vi "TCP Send Synchronous Request.vi"(8 "error in (no error)":errorcluster, 10 "Request String in":string) -> (0 "error out":errorcluster, 2 "Response":string)   [LabVIEW 2015]
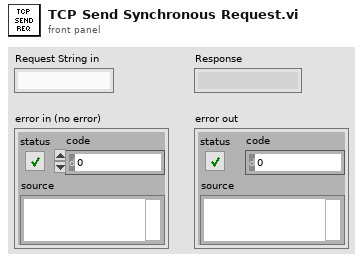
[diagram p1: front panel]
types:
  T1 = enum16{"Standard", "Buffered", "CRLF", "Immediate"}
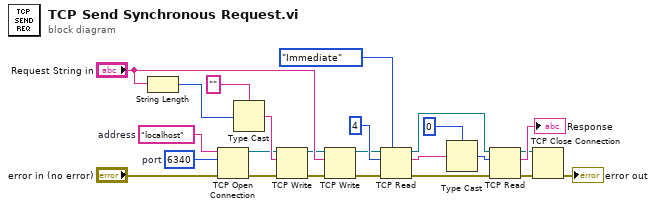
[diagram p0: block diagram]
diagram:
  w3 = u16 6340  # port
  w2 = "localhost"  # address
  n1 = String Length(string="Request String in") -> (length=w12:i32)
  n2 = TCP Open Connection(address=w2, remote port or service name=w3, error in (no error)="error in (no error)") -> (connection ID=w7:refnum<k5>, error out=w9:errorcluster)  [unwired: 2 in]
  n3 = Type Cast(type="" ("format string"), x=w12) -> (*(type *) &x=w11:string)
  n4 = TCP Write(connection ID=w7, data in=w11, error in (no error)=w9) -> (connection ID out=w8:refnum<k5>, error out=w10:errorcluster)  [unwired: 1 in, 1 out]
  n5 = TCP Write(connection ID=w8, data in="Request String in", error in (no error)=w10) -> (connection ID out=w4:refnum<k5>, error out=w5:errorcluster)  [unwired: 1 in, 1 out]
  n6 = TCP Read(connection ID=w4, bytes to read=4, error in (no error)=w5, 7:T1."Immediate" ("mode (standard)")) -> (connection ID out=w20:refnum<k5>, data out=w16:string, error out=w18:errorcluster)  [unwired: 1 in]
  n7 = Type Cast(type=0 ("bytes to read"), x=w16) -> (*(type *) &x=w17:i32)
  n8 = TCP Read(connection ID=w20, bytes to read=w17, error in (no error)=w18) -> (connection ID out=w21:refnum<k5>, data out=→"Response":string, error out=w19:errorcluster)  [unwired: 2 in]
  n9 = TCP Close Connection(connection ID=w21, error in (no error)=w19) -> (error out=→"error out":errorcluster)  [unwired: 1 in, 1 out]
